vi "Unit Tests.vi"   [LabVIEW 2020]
uses:
  <vilib>/addons/_JKI Toolkits/Caraya/classes/Test/Test.lvclass
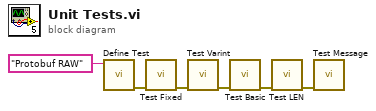
[diagram p0: block diagram]
diagram:
  n1 = call <vilib>:"Define Test.vi"("Label (VI Title)"="Protobuf RAW") -> ("error out"=w2:errorcluster)  [unwired: 10 in]
  n2 = call "Test Fixed.vi"("error in (no error)"=w2) -> ("error out"=w1:errorcluster)  [unwired: 10 in]
  n3 = call "Test Varint.vi"("error in (no error)"=w1) -> ("error out"=w5:errorcluster)  [unwired: 10 in]
  n4 = call "Test Basic.vi"("error in (no error)"=w5) -> ("error out"=w4:errorcluster)  [unwired: 10 in]
  n5 = call "Test LEN.vi"("error in (no error)"=w4) -> ("error out"=w3:errorcluster)  [unwired: 10 in]
  n6 = call "Test Message.vi"("error in (no error)"=w3) -> ()  [unwired: 10 in, 1 out]
